vi "Dynamic Wrapper.vi"(8 "error in (no error)":errorcluster, 11 "Test Class in":refnum<class "Test Class.lvclass">) -> (0 "error out":errorcluster, 3 "Test Class out":refnum<class "Test Class.lvclass">)   [LabVIEW 2024, in "Test Class.lvclass"]
uses:
  Test Class.lvclass
  Test Class.lvclass/Test Class.ctl
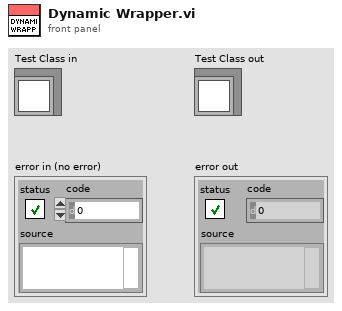
[diagram p1: front panel]
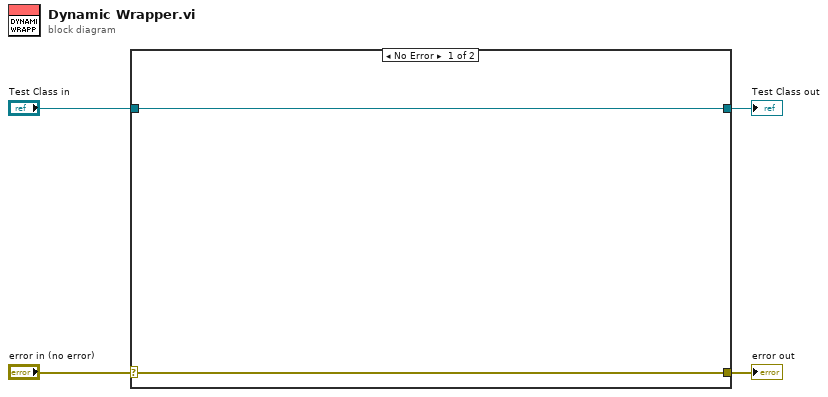
[diagram p0: block diagram]
diagram:
  n1 = case shown="No Error" "error in (no error)" {
    selector: "error in (no error)" -> [w5 w8]
    tunnel: [w5 w8] -> w3
    tunnel: [w6 w7] -> w1
    tunnel: "Test Class in" -> [w6 w7]
    frame No Error {
    }
    frame Error {
    }
  }
  "error out" <- w3
  "Test Class out" <- w1
